vi "RT_NetStreams.vi"() -> ()   [LabVIEW 2019]
panel:
  out "Waveform Chart":dbl(graph)
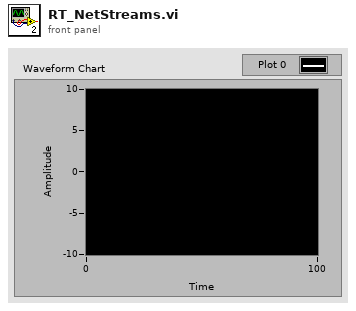
[diagram p1: front panel]
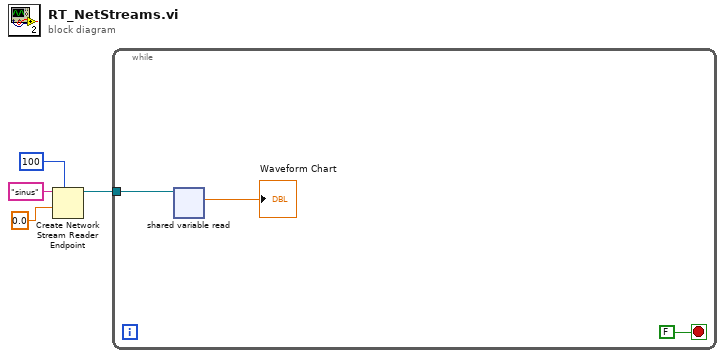
[diagram p0: block diagram]
diagram:
  n1 = Create Network Stream Reader Endpoint(7:100 ("reader buffer size"), 9:0.0, 11:"sinus" ("reader name")) -> (3:w1:refnum<k21>)  [unwired: 4 in, 1 out]
  n2 = while {
    tunnel: w1 -> [w7]
    stop <- FALSE stop-if-true
    n3 = shared-variable-read(w7) -> (→"Waveform Chart":dbl)  [unwired: 2 in, 3 out]
  }
